vi "6. Module Attributes.vi"() -> ()   [LabVIEW 2017]
doc: "### 6. Module Attributes.vi\n\n#### Overview\n\nDemonstrates how to dynamically interact with CSM module attributes using VIs from outside the CSM framework.\n\n#### Introduction\n\nThis example demonstrates how to dynamically interact with CSM module attributes using VIs from outside the CSM framework.\n\nThe following are three ways of interaction within CSM framework:\n\n- Use string message queue to transfer message locally/outside of CSM framework, such as State >> Argument -@ DestModuleName.\n- Broadcast/Interrupt a status change event from a CSM module, register/unregister that event from another CSM/non-CSM module.\n- Use Module Attribute related VIs to get/set/remove/list CSM module attributes.\n\nThe core function of this example is from outside the CSM module to dynamically set another random number value to the CSM module, and then get the value from the CSM module and display the value on the UI.\n\n#### Steps\n\nStep 1: Drop the VI template from LabVIEW CSM palette.\n\nStep 2: Add one new line of state string after Macro:Initialize, namely API: Define ABC Attribute.\n\nStep 3: Set Module Attribute inside the CSM module: abc as attribute, a random number as value.\n\nStep 4: Set Module Attribute from outside the CSM module: abc as attribute, a random number as value.\n\nStep 5: Set Module Attribute from outside the CSM module: abc as attribute, retrieve the set random number as value.\n\nStep 6: Send a synchronous message to stop the CSM module from outside the CSM module."
uses:
  user.lib/_NEVSTOP/Communicable State Machine(CSM)/AdvanceAPI/CSM - Revert Arguments-Safe String.vi
  user.lib/_NEVSTOP/Communicable State Machine(CSM)/AdvanceAPI/CSM - Make String Arguments Safe.vi
  user.lib/_NEVSTOP/Communicable State Machine(CSM)/AdvanceAPI/CSM - Break Down Multiple States String.vi
  user.lib/_NEVSTOP/Communicable State Machine(CSM)/AdvanceAPI/CSM - Compact Multiple States.vi
  user.lib/_NEVSTOP/Communicable State Machine(CSM)/AdvanceAPI/CSM - Keywords.vi
  user.lib/_NEVSTOP/Communicable State Machine(CSM)/_Shared/Trim Single-line Text.vi
  user.lib/_NEVSTOP/Communicable State Machine(CSM)/Communicable State Machine.lvlib
panel:
  out "Waited(ms) 2":u32
  out "Waited(ms)":u32
  out "error out":errorcluster
  out "abc":dbl
  out "State History":string
  # "#CSM-Example Overview\n\nDemonstrates how to dynamically interact with CSM module attributes using VIs from outside the CSM framework."
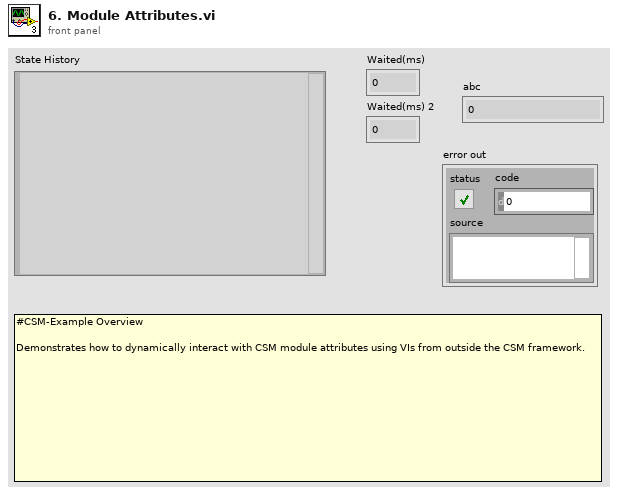
[diagram p1: front panel]
types:
  T1 = enum32{"Invalid", "Standard", "Closed", "Hidden", "Minimized", "Maximized"}
  T2 = enum32{"invalid app kind", "Development System", "Run Time System", "Student Edition", "Embedded LabVIEW", "Evaluation", "Custom"}
  T3 = typedef "Communicable State Machine.lvlib/_CSM_Response Source Message.ctl" = cluster{"‘State":string, "’Arguments":string, "’Error":errorcluster}
  T4 = cluster{"Current VI Reference":refnum<vi>, "Close Panel on Exit?":bool}
  T5 = cluster{"Core":cluster{"Current VI Reference":refnum<vi>, "Close Panel on Exit?":bool}, "Your Boolean data":bool, "Your string data":string}
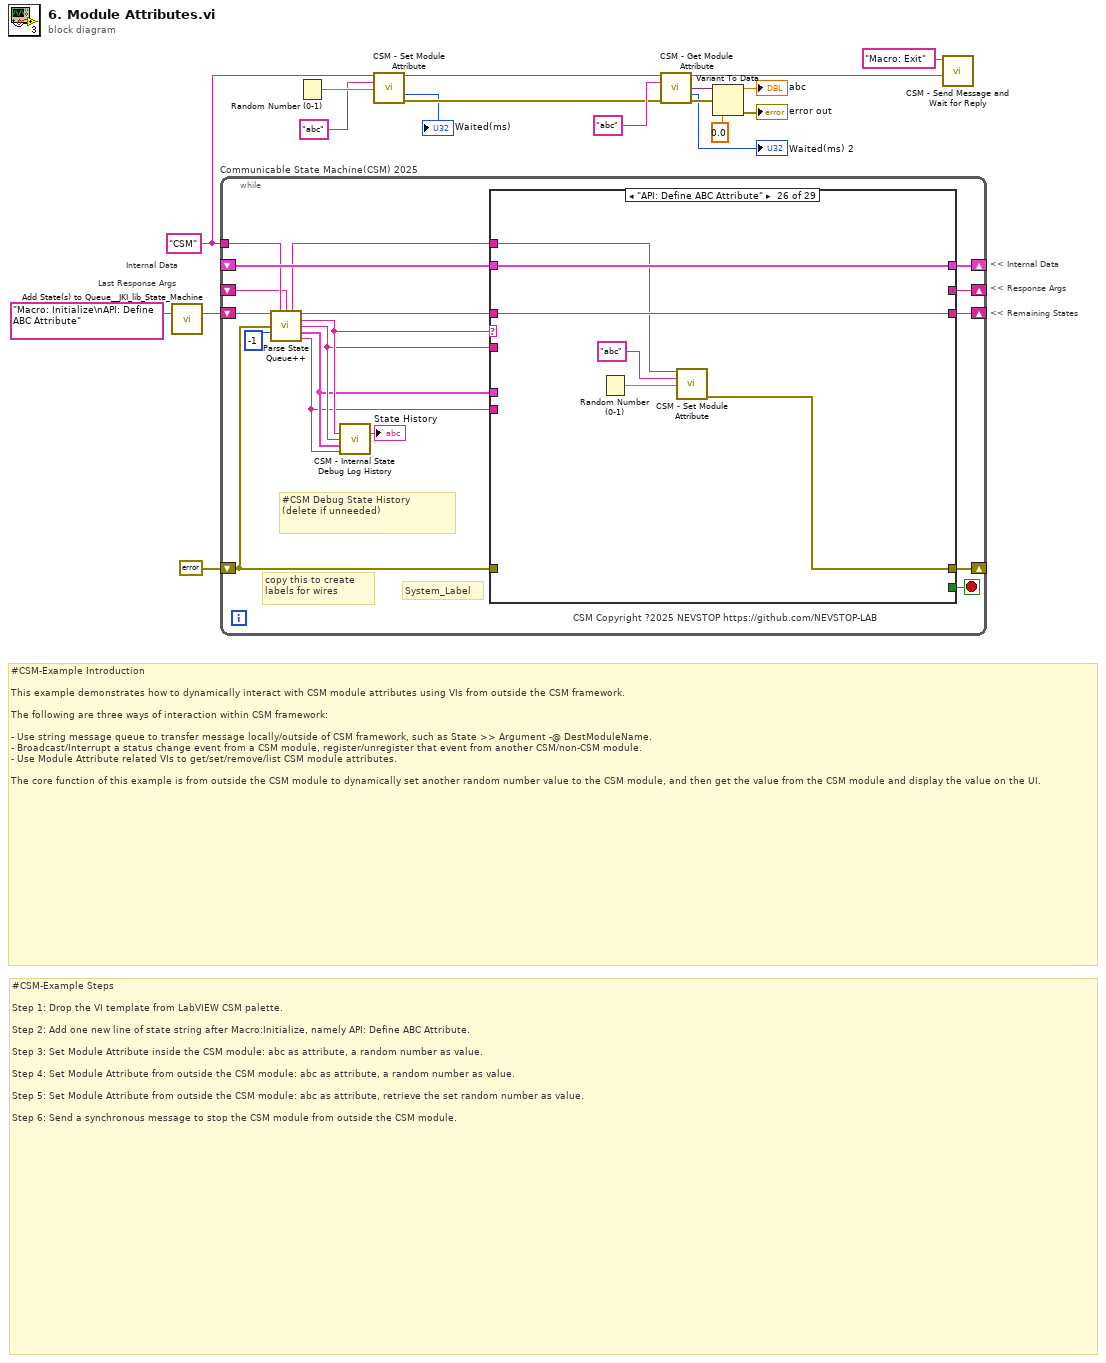
[diagram p0: block diagram]
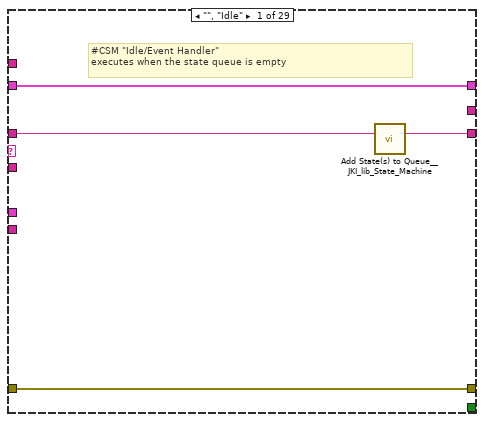
[diagram p2: hidden frame]
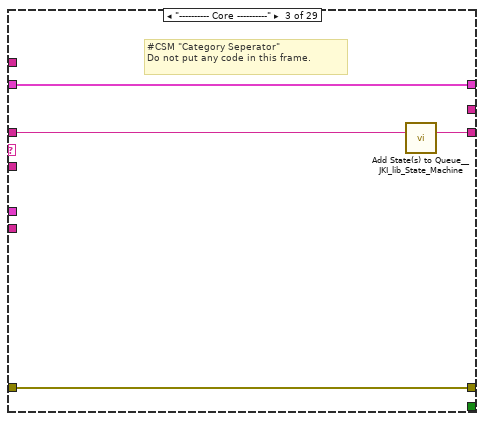
[diagram p4: hidden frame]
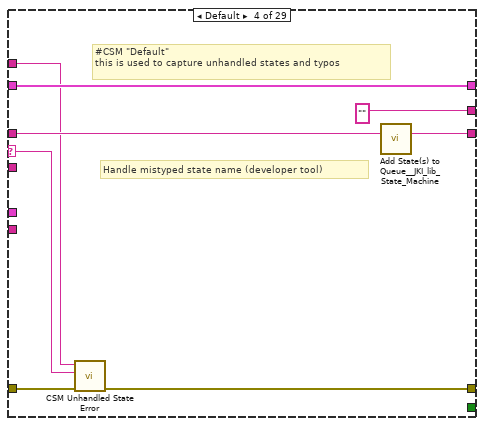
[diagram p5: hidden frame]
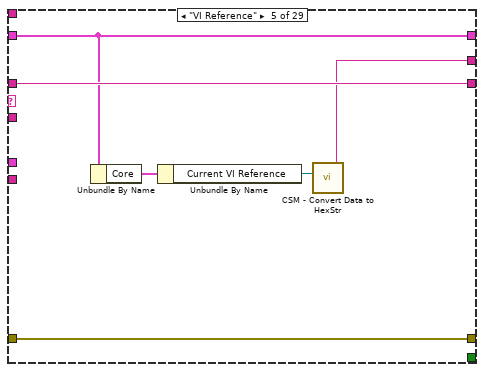
[diagram p6: hidden frame]
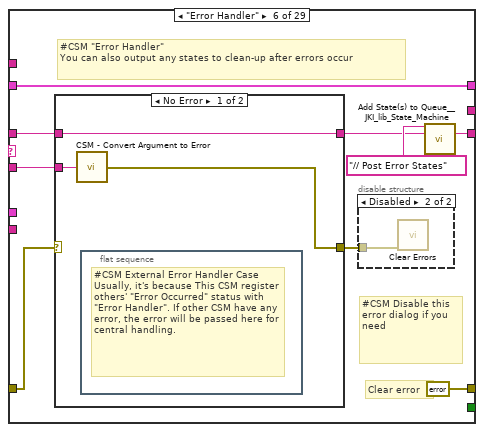
[diagram p7: hidden frame]
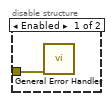
[diagram p8: hidden frame]
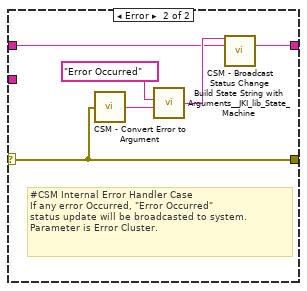
[diagram p9: hidden frame]
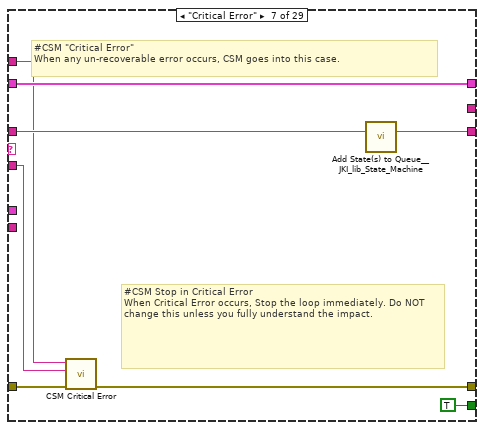
[diagram p10: hidden frame]
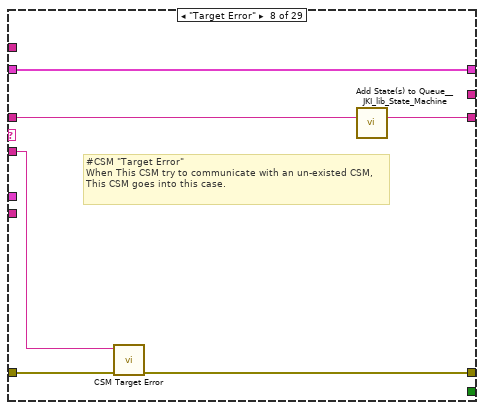
[diagram p11: hidden frame]
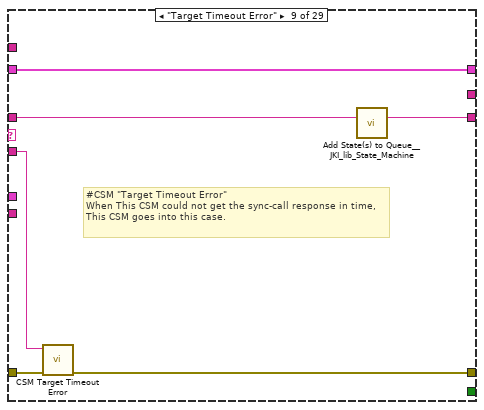
[diagram p12: hidden frame]
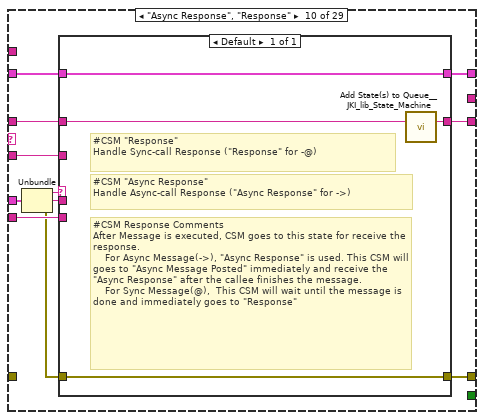
[diagram p13: hidden frame]
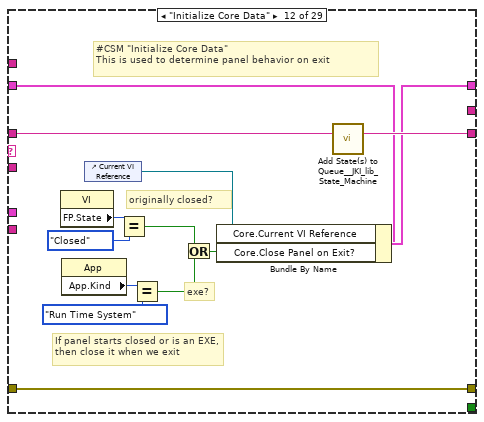
[diagram p15: hidden frame]
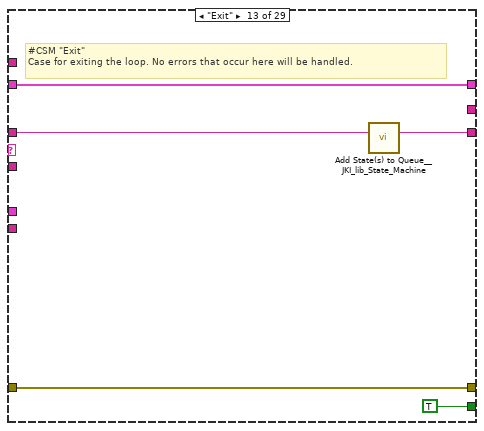
[diagram p16: hidden frame]
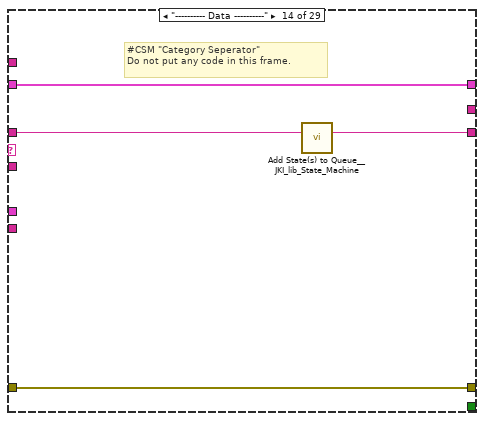
[diagram p17: hidden frame]
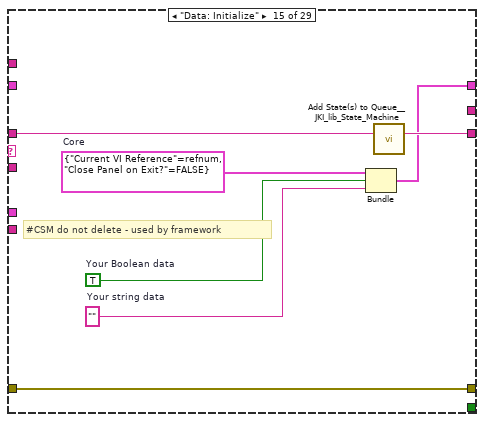
[diagram p18: hidden frame]
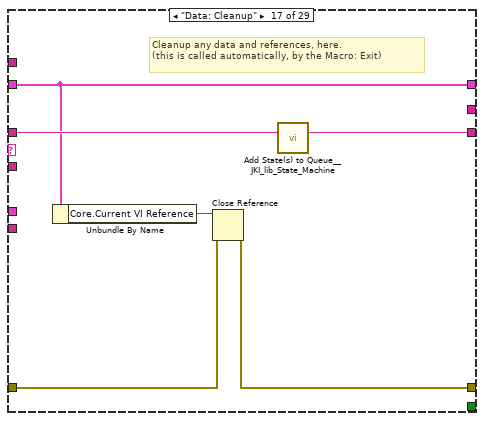
[diagram p20: hidden frame]
diagram:
  w3 = "CSM" ("Name(\"\" to use uuid)")
  # "#CSM-Example Steps\n\nStep 1: Drop the VI template from LabVIEW CSM palette.\n\nStep 2: Add one new line of state string after Macro:Initialize, namely API: Define ABC Attribute.\n\nStep 3: Set Module Attribute inside the CSM module: abc as attribute, a random number as value.\n\nStep 4: Set Module Attribute from outside the CSM module: abc as attribute, a random number as value.\n\nStep 5: Set Module Attribute from outside the CSM module: abc as attribute, retrieve the set random number as value.\n\nStep 6: Send a synchronous message to stop the CSM module from outside the CSM module."
  # "#CSM-Example Introduction\n\nThis example demonstrates how to dynamically interact with CSM module attributes using VIs from outside the CSM framework.\n\nThe following are three ways of interaction within CSM framework:\n\n- Use string message queue to transfer message locally/outside of CSM framework, such as State >> Argument -@ DestModuleName.\n- Broadcast/Interrupt a status change event from a CSM module, register/unregister that event from another CSM/non-CSM module.\n- Use Module Attribute related VIs to get/set/remove/list CSM module attributes.\n\nThe core function of this example is from outside the CSM module to dynamically set another random number value to the CSM module, and then get the value from the CSM module and display the value on the UI."
  # "Last Response Args"
  # "Internal Data"
  # "<< Internal Data"
  # "<< Response Args"
  # "<< Remaining States"
  n1 = call <vilib>:"Add State(s) to Queue__JKI_lib_State_Machine.vi"("State(s) in (\"\")"="Macro: Initialize\nAPI: Define ABC Attribute" ("Init State(\"Macro: Initialize\")")) -> ("States Out"=w16:string)  [unwired: 14 in]
  n2 = while "Communicable State Machine(CSM) 2025" {
    shift-right: [w31] -> _
    shift-left: _ -> [w30]
    shift-right: [w34] -> _
    shift-left: errorcluster {"status"=FALSE, "code"=0, "source"=""} ("error out") -> [w29]
    shift-right: [w33] -> _
    shift-left: w16 -> [w35]
    tunnel: w3 -> [w27]
    shift-right: [w28] -> _
    shift-left: _ -> [w21]
    stop <- w32 stop-if-true
    # "#CSM Debug State History\n(delete if unneeded)"
    # "copy this to create labels for wires"
    # "System_Label"
    # "CSM Copyright ?2025 NEVSTOP https://github.com/NEVSTOP-LAB"
    n3 = call "Parse State Queue++.vi"("State Queue"=w35, "Name (\"\" to Use UUID)"=w27, "Response Arguments"=w21, "Previous Error"=w29, "Dequeue (1 ms)"=-1 ("Timeout")) -> ("Name Used"=w22:string, "Remaining States"=w36:string, "Current State"=w26:string, "Arguments"=w25:string, ">> Response Source Message >>"=w24:T3, ">> Source CSM >>"=w23:string)  [unwired: 5 in]
    n4 = call "CSM - Internal State Debug Log History.vi"("State"=w26, "Arguments (\"\")"=w25, ">> Response Source Message >>"=w24, "Source (\"\")"=w23) -> ("Debug Log"=→"State History":string)  [unwired: 11 in]
    n5 = case shown="\"API: Define ABC Attribute\"" w26 {
      selector: w26 -> [_ _ _ w50 _ _ _ _ _ _ _ _ _ _ _ _ _ _ _ _ _ _ _ _ _ _ _ _ _]
      tunnel: w36 -> [w37 w42 w47 w54 w60 w66 w87 w93 w99 w107 w118 w132 w137 w141 w148 w150 w157 w161 w165 w171 w186 w255 w260 w267 w269 w276 w280 w284 w288]
      tunnel: w25 -> [_ _ _ _ _ w65 w83 w92 w97 w106 _ _ _ _ _ _ _ _ _ w166 w180 _ _ _ _ _ _ _ _]
      tunnel: w30 -> [w38 w41 w44 w52 w59 w69 w88 w94 w100 w109 w117 w125 w135 w138 _ w149 w152 w158 w163 w169 w182 w252 w257 w264 w268 w275 w277 w281 w285]
      tunnel: [w39 w43 w45 w48 w61 errorcluster {"status"=FALSE, "code"=0, "source"=""} ("error out") w84 w90 w96 w112 w119 w129 w134 w139 w145 w151 w153 w159 w162 w167 w183 w253 w258 w265 w270 w271 w278 w282 w286] -> w34
      tunnel: w29 -> [w39 w43 w45 w55 w61 w67 w89 w91 w98 _ w119 w129 w134 w139 w145 w151 w154 w159 w162 w168 w184 w253 w258 w265 w270 _ w278 w282 w286]
      tunnel: [w40 w42 w46 w53 w60 w62 w86 w95 w101 w108 w118 w131 w136 w140 w147 w150 w156 w160 w164 w170 w185 w254 w259 w266 w269 w276 w279 w283 w287] -> w33
      tunnel: [_ _ _ _ _ _ TRUE _ _ _ _ _ TRUE _ _ _ _ _ _ _ _ _ _ _ _ _ _ _ _] -> w32
      tunnel: [w38 w41 w44 w52 w59 w69 w88 w94 w100 w110 w117 w130 w135 w138 w146 w149 w152 w158 w163 w169 w182 w252 w257 w264 w268 w275 w277 w281 w285] -> w31
      tunnel: w23 -> [_ _ _ _ _ _ _ _ _ w104 _ _ _ _ _ _ _ _ _ _ _ _ _ _ _ _ _ _ _]
      tunnel: w24 -> [_ _ _ _ _ _ _ _ _ w111 _ _ _ _ _ _ _ _ _ _ _ _ _ _ _ _ _ _ _]
      tunnel: [_ _ _ "" w56 _ _ _ _ _ _ _ _ _ _ _ _ _ _ _ _ _ _ _ _ _ _ _ _] -> w28
      tunnel: w22 -> [_ _ _ w49 _ _ w82 _ _ _ _ _ _ _ _ _ _ _ _ _ _ _ _ _ _ w272 _ _ _]
      frame "", "Idle" {
        # "#CSM \"Idle/Event Handler\"\nexecutes when the state queue is empty"
        n6 = call <vilib>:"Add State(s) to Queue__JKI_lib_State_Machine.vi"("State(s) in (\"\")"=w37) -> ("States Out"=w40:string)  [unwired: 14 in]
      }
      frame "CSM Documentation" {
        # "#CSM README FIRST\n\nCommunicable State Machine(CSM) is a LabVIEW application framework that builds upon JKI State Machine(JKISM). It follows the pattern of JKISM and extends the keywords to describe message communication between modules, including concepts such as Sync-Message, Async-Message, Subscription/Unsubscription of status - essential elements for creating reusable code modules. For more information, please visit the CSM wiki: https://nevstop-lab.github.io/CSM-Wiki/\n\nFor instructions on JKI State Machine, visit: http://jki.net/state-machine/\nFor information about CSM, visit: https://github.com/NEVSTOP-LAB"
        # "#CSM \"Documentation\"\nCase for holding CSM Documenation"
      }
      frame "---------- Core ----------" {
        # "#CSM \"Category Seperator\"\nDo not put any code in this frame."
        n7 = call <vilib>:"Add State(s) to Queue__JKI_lib_State_Machine.vi"("State(s) in (\"\")"=w47) -> ("States Out"=w46:string)  [unwired: 14 in]
      }
      frame Default {
        # "#CSM \"Default\"\nthis is used to capture unhandled states and typos"
        # "Handle mistyped state name (developer tool)"
        n8 = call "CSM Unhandled State Error.vi"("error in (no error)"=w55, "Current State"=w50, "CSM Name"=w49) -> ("error out"=w48:errorcluster)  [unwired: 8 in]
        n9 = call <vilib>:"Add State(s) to Queue__JKI_lib_State_Machine.vi"("State(s) in (\"\")"=w54) -> ("States Out"=w53:string)  [unwired: 14 in]
      }
      frame "VI Reference" {
        n10 = Unbundle By Name(w59) -> ("Core"=w58:T4)
        n11 = Unbundle By Name(w58) -> ("Current VI Reference"=w57:refnum<vi>)
        n12 = call "CSM - Convert Data to HexStr.vi"("Variant"=w57) -> ("HEX String (0-9,A-F)"=w56:string)  [unwired: 8 in]
      }
      frame "Error Handler" {
        # "#CSM Disable this error dialog if you need"
        # "#CSM \"Error Handler\"\nYou can also output any states to clean-up after errors occur"
        # "Clear error"
        n13 = case shown="No Error" w67 {
          selector: w67 -> [_ w76]
          tunnel: [w75 w78] -> w63
          tunnel: w66 -> [w75 w77]
          tunnel: w65 -> [w74 _]
          tunnel: [w73 w76] -> w68
          frame No Error {
            n14 = call "CSM - Convert Argument to Error.vi"("Argument"=w74) -> ("Error"=w73:errorcluster)  [unwired: 4 in]
            n15 = flat-sequence {
              frame #0 {
                # "#CSM External Error Handler Case\nUsually, it's because This CSM register others' \"Error Occurred\" status with \"Error Handler\". If other CSM have any error, the error will be passed here for central handling."
              }
            }
          }
          frame Error {
            # "#CSM Internal Error Handler Case \nIf any error Occurred, \"Error Occurred\" \nstatus update will be broadcasted to system.\nParameter is Error Cluster."
            n16 = call "CSM - Convert Error to Argument.vi"("Error"=w76) -> ("Argument"=w80:string)  [unwired: 4 in]
            n17 = call <vilib>:"Build State String with Arguments__JKI_lib_State_Machine.vi"("Arguments (\"\")"=w80, "State"="Error Occurred" ("Status with Arguments")) -> ("State with Arguments"=w79:string)  [unwired: 4 in]
            n18 = call "CSM - Broadcast Status Change.vi"("Status With Arguments"=w79, "State Queue"=w77) -> ("Remaining States"=w78:string)  [unwired: 13 in]
          }
        }
        n19 = disable-structure shown="Disabled" {
          disable-tunnel: w68 -> [w71 w72]
          frame Enabled {
            n20 = call <vilib>:"General Error Handler.vi"("error in (no error)"=w71) -> ()  [unwired: 10 in, 5 out]
          }
          frame Disabled {
            n21 = call <vilib>:"Clear Errors.vi"("error in (no error)"=w72) -> ()  [unwired: 5 in, 2 out]
          }
        }
        n22 = call <vilib>:"Add State(s) to Queue__JKI_lib_State_Machine.vi"("State(s) in Front (\"\")"="// Post Error States", "State(s) in (\"\")"=w63) -> ("States Out"=w62:string)  [unwired: 13 in]
      }
      frame "Critical Error" {
        # "#CSM Stop in Critical Error\nWhen Critical Error occurs, Stop the loop immediately. Do NOT change this unless you fully understand the impact."
        # "#CSM \"Critical Error\"\nWhen any un-recoverable error occurs, CSM goes into this case."
        n23 = call "CSM Critical Error.vi"("error in (no error)"=w89, "Arugments (As Reason)"=w83, "CSM Name"=w82) -> ("error out"=w84:errorcluster)  [unwired: 8 in]
        n24 = call <vilib>:"Add State(s) to Queue__JKI_lib_State_Machine.vi"("State(s) in (\"\")"=w87) -> ("States Out"=w86:string)  [unwired: 14 in]
      }
      frame "Target Error" {
        # "#CSM \"Target Error\"\nWhen This CSM try to communicate with an un-existed CSM, This CSM goes into this case."
        n25 = call "CSM Target Error.vi"("error in (no error)"=w91, "Arguments (As CSM Name)"=w92) -> ("error out"=w90:errorcluster)  [unwired: 9 in]
        n26 = call <vilib>:"Add State(s) to Queue__JKI_lib_State_Machine.vi"("State(s) in (\"\")"=w93) -> ("States Out"=w95:string)  [unwired: 14 in]
      }
      frame "Target Timeout Error" {
        # "#CSM \"Target Timeout Error\"\nWhen This CSM could not get the sync-call response in time, This CSM goes into this case."
        n27 = call "CSM Target Timeout Error.vi"("error in (no error)"=w98, "Arguments (As CSM Name)"=w97) -> ("error out"=w96:errorcluster)  [unwired: 9 in]
        n28 = call <vilib>:"Add State(s) to Queue__JKI_lib_State_Machine.vi"("State(s) in (\"\")"=w99) -> ("States Out"=w101:string)  [unwired: 14 in]
      }
      frame "Async Response", "Response" {
        n29 = Unbundle(w111) -> ("‘State"=w105:string, "’Arguments"=w103:string, "’Error"=w102:errorcluster)
        n30 = case shown="Default" w105 {
          tunnel: [w116] -> w112
          tunnel: w102 -> [w116]
          tunnel: [w115] -> w110
          tunnel: w109 -> [w115]
          tunnel: [w113] -> w108
          tunnel: w107 -> [w114]
          tunnel: w106 -> [_]
          tunnel: w104 -> [_]
          tunnel: w103 -> [_]
          frame Default {
            # "#CSM Response Comments\nAfter Message is executed, CSM goes to this state for receive the response.\n    For Async Message(->), \"Async Response\" is used. This CSM will goes to \"Async Message Posted\" immediately and receive the \"Async Response\" after the callee finishes the message.\n    For Sync Message(@),  This CSM will wait until the message is done and immediately goes to \"Response\""
            # "#CSM \"Async Response\"\nHandle Async-call Response (\"Async Response\" for ->)"
            # "#CSM \"Response\"\nHandle Sync-call Response (\"Response\" for -@)"
            n31 = call <vilib>:"Add State(s) to Queue__JKI_lib_State_Machine.vi"("State(s) in (\"\")"=w114) -> ("States Out"=w113:string)  [unwired: 14 in]
          }
        }
      }
      frame "Async Message Posted" {
        # "#CSM \"Async Message Posted\"\nAfter Async Message is posted (-> or ->| ), CSM goes to this state for post-action.\nYou can use Argument - State to tell which Async Message is called."
      }
      frame "Initialize Core Data" {
        # "#CSM \"Initialize Core Data\"\nThis is used to determine panel behavior on exit"
        # "originally closed?"
        # "exe?"
        # "If panel starts closed or is an EXE, then close it when we exit"
        n32 = property class="VI"() -> ("FP.State"=w122:T1)  [unwired: 2 in, 2 out]
        n33 = property class="App"() -> ("App.Kind"=w128:T2)  [unwired: 2 in, 2 out]
        n34 = control-ref of="Current VI Reference"() -> (w123:refnum<vi>)
        n35 = Equal?(x=w122, y=T1."Closed" ("Front Panel Window:State")) -> (x = y?=w120:bool)
        n36 = Equal?(x=w128, y=T2."Run Time System" ("Application:Kind")) -> (x = y?=w126:bool)
        n37 = Or(x=w120, y=w126) -> (x .or. y?=w124:bool)
        n38 = Bundle By Name(cluster=w125, "Core.Current VI Reference"=w123, "Core.Close Panel on Exit?"=w124) -> (w130:T5)
        n39 = call <vilib>:"Add State(s) to Queue__JKI_lib_State_Machine.vi"("State(s) in (\"\")"=w132) -> ("States Out"=w131:string)  [unwired: 14 in]
      }
      frame "Exit" {
        # "#CSM \"Exit\"\nCase for exiting the loop. No errors that occur here will be handled."
        n40 = call <vilib>:"Add State(s) to Queue__JKI_lib_State_Machine.vi"("State(s) in (\"\")"=w137) -> ("States Out"=w136:string)  [unwired: 14 in]
      }
      frame "---------- Data ----------" {
        # "#CSM \"Category Seperator\"\nDo not put any code in this frame."
        n41 = call <vilib>:"Add State(s) to Queue__JKI_lib_State_Machine.vi"("State(s) in (\"\")"=w141) -> ("States Out"=w140:string)  [unwired: 14 in]
      }
      frame "Data: Initialize" {
        w142 = T4 {"Current VI Reference"=refnum, "Close Panel on Exit?"=FALSE}  # Core
        w144 = TRUE  # Your Boolean data
        w143 = ""  # Your string data
        # "#CSM do not delete - used by framework"
        n42 = Bundle("Core"=w142, "Your Boolean data"=w144, "Your string data"=w143) -> (w146:T5)  [unwired: 1 in]
        n43 = call <vilib>:"Add State(s) to Queue__JKI_lib_State_Machine.vi"("State(s) in (\"\")"=w148) -> ("States Out"=w147:string)  [unwired: 14 in]
      }
      frame "Data: Update Indicators" {
      }
      frame "Data: Cleanup" {
        # "Cleanup any data and references, here.\n(this is called automatically, by the Macro: Exit)"
        n44 = Unbundle By Name(w152) -> ("Core.Current VI Reference"=w155:refnum<vi>)
        n45 = Close Reference(reference=w155, error in (no error)=w154) -> (error out=w153:errorcluster)
        n46 = call <vilib>:"Add State(s) to Queue__JKI_lib_State_Machine.vi"("State(s) in (\"\")"=w157) -> ("States Out"=w156:string)  [unwired: 14 in]
      }
      frame "---------- UI ----------" {
        # "#CSM \"Category Seperator\"\nDo not put any code in this frame."
        n47 = call <vilib>:"Add State(s) to Queue__JKI_lib_State_Machine.vi"("State(s) in (\"\")"=w161) -> ("States Out"=w160:string)  [unwired: 14 in]
      }
      frame "UI: Initialize" {
        # "#CSM \"UI: Initialize\"\nInitialize the User Interface, here.\n(this is called automatically, by the Macro: Init)"
        n48 = call <vilib>:"Add State(s) to Queue__JKI_lib_State_Machine.vi"("State(s) in (\"\")"=w165) -> ("States Out"=w164:string)  [unwired: 14 in]
      }
      frame "UI: Cursor Set" {
        # "#CSM \"UI: Cursor Set\"\nSet and Unset Cursor Busy.\n(Usage: \"UI: Cursor Set >> Busy|Idle\")"
        # "Argument"
        n49 = disable-structure shown="TARGET_TYPE!=Windows" {
          disable-tunnel: w168 -> [w174 w179]
          disable-tunnel: [w173 w179] -> w167
          disable-tunnel: w166 -> [w172 _]
          frame condition #0 (active) {
            n50 = case shown="\"Idle\", Default" w172 {
              tunnel: w174 -> [w176 w178]
              tunnel: [w175 w177] -> w173
              frame "Idle", Default {
                n51 = call <vilib>:"Unset Busy.vi"("error in (no error)"=w176) -> ("error out"=w175:errorcluster)  [unwired: 10 in]
              }
              frame "Busy" {
                n52 = call <vilib>:"Set Busy.vi"("error in (no error)"=w178) -> ("error out"=w177:errorcluster)  [unwired: 9 in, 1 out]
              }
            }
          }
          frame condition #1 {
          }
        }
        n53 = call <vilib>:"Add State(s) to Queue__JKI_lib_State_Machine.vi"("State(s) in (\"\")"=w171) -> ("States Out"=w170:string)  [unwired: 14 in]
      }
      frame "UI: Front Panel State" {
        # "#CSM \"UI: Front Panel State\"\nSet Front Panel Open or Closed\n(Usage: \"UI: Front Panel State >> Open|Close\")"
        # "Argument"
        n54 = Unbundle By Name(w182) -> ("Core.Current VI Reference"=w181:refnum<vi>)
        n55 = call <vilib>:"Add State(s) to Queue__JKI_lib_State_Machine.vi"("State(s) in (\"\")"=w186) -> ("States Out"=w185:string)  [unwired: 14 in]
        n56 = case shown="\"Close\", \"Closed\"" w180 {
          tunnel: w184 -> [w192 w207 w218 w231 w244]
          tunnel: [w194 w208 w220 w233 w246] -> w183
          tunnel: w181 -> [w193 w205 w219 w232 w245]
          frame "Open", "Standard", Default {
            w187 = T1."Standard" ("State")
            n57 = property class="VI"(reference=w193, error in=w192) -> (reference out=w190:refnum<vi>, error out=w191:errorcluster, "FP.State"=w189:T1)
            n58 = Not Equal?(x=w189, y=w187) -> (x != y?=w188:bool)
            n59 = case shown="True" w188 {
              tunnel: [w198 w200] -> w194
              tunnel: w191 -> [w197 w200]
              tunnel: w190 -> [w196 _]
              tunnel: w187 -> [w195 _]
              frame True {
                n60 = invoke class="VI" method="FP.Open"(reference=w196, error in=w197, "Activate"=TRUE, "State"=w195) -> (error out=w198:errorcluster)  [unwired: 1 in, 4 out]
              }
              frame False {
              }
            }
          }
          frame "Close", "Closed" {
            n61 = property class="VI"(reference=w205, error in=w207) -> (reference out=w204:refnum<vi>, error out=w206:errorcluster, "FP.State"=w202:T1)
            n62 = Not Equal?(x=w202, y=T1."Closed" ("Front Panel Window:State")) -> (x != y?=w201:bool)
            n63 = case shown="False" w201 {
              tunnel: [w209 w212] -> w208
              tunnel: w206 -> [w209 w211]
              tunnel: w204 -> [_ w210]
              frame False {
              }
              frame True {
                n64 = invoke class="VI" method="FP.Close"(reference=w210, error in=w211) -> (error out=w212:errorcluster)  [unwired: 1 in, 2 out]
              }
            }
          }
          frame "Hidden", "Hide" {
            w213 = T1."Hidden" ("State")
            n65 = property class="VI"(reference=w219, error in=w218) -> (reference out=w216:refnum<vi>, error out=w217:errorcluster, "FP.State"=w215:T1)
            n66 = Not Equal?(x=w215, y=w213) -> (x != y?=w214:bool)
            n67 = case shown="True" w214 {
              tunnel: [w224 w225] -> w220
              tunnel: w217 -> [w223 w225]
              tunnel: w216 -> [w222 _]
              tunnel: w213 -> [w221 _]
              frame True {
                n68 = invoke class="VI" method="FP.Open"(reference=w222, error in=w223, "State"=w221) -> (error out=w224:errorcluster)  [unwired: 2 in, 4 out]
              }
              frame False {
              }
            }
          }
          frame "Minimize", "Minimized" {
            w226 = T1."Minimized" ("State")
            n69 = property class="VI"(reference=w232, error in=w231) -> (reference out=w229:refnum<vi>, error out=w230:errorcluster, "FP.State"=w228:T1)
            n70 = Not Equal?(x=w228, y=w226) -> (x != y?=w227:bool)
            n71 = case shown="True" w227 {
              tunnel: [w237 w238] -> w233
              tunnel: w230 -> [w236 w238]
              tunnel: w229 -> [w235 _]
              tunnel: w226 -> [w234 _]
              frame True {
                n72 = invoke class="VI" method="FP.Open"(reference=w235, error in=w236, "State"=w234) -> (error out=w237:errorcluster)  [unwired: 2 in, 4 out]
              }
              frame False {
              }
            }
          }
          frame "Maximize", "Maximized" {
            w239 = T1."Maximized" ("State")
            n73 = property class="VI"(reference=w245, error in=w244) -> (reference out=w242:refnum<vi>, error out=w243:errorcluster, "FP.State"=w241:T1)
            n74 = Not Equal?(x=w241, y=w239) -> (x != y?=w240:bool)
            n75 = case shown="True" w240 {
              tunnel: [w250 w251] -> w246
              tunnel: w243 -> [w249 w251]
              tunnel: w242 -> [w248 _]
              tunnel: w239 -> [w247 _]
              frame True {
                n76 = invoke class="VI" method="FP.Open"(reference=w248, error in=w249, "State"=w247) -> (error out=w250:errorcluster)  [unwired: 2 in, 4 out]
              }
              frame False {
              }
            }
          }
        }
      }
      frame "---------- Macro ----------" {
        # "#CSM \"Category Seperator\"\nDo not put any code in this frame."
        n77 = call <vilib>:"Add State(s) to Queue__JKI_lib_State_Machine.vi"("State(s) in (\"\")"=w255) -> ("States Out"=w254:string)  [unwired: 14 in]
      }
      frame "Macro: Initialize" {
        # "#CSM \"Macro: Initialize\"\nInitialization Macro (This is called once, when the VI starts)"
        n78 = call <vilib>:"Add State(s) to Queue__JKI_lib_State_Machine.vi"("State(s) in Front (\"\")"="Data: Initialize\nInitialize Core Data\nData: Update Indicators", "State(s) in (\"\")"=w260) -> ("States Out"=w259:string)  [unwired: 13 in]
      }
      frame "Macro: Exit" {
        # "#CSM \"Macro: Exit\"\nExit Macro (This is called once, when the VI exits)"
        n79 = call <vilib>:"Add State(s) to Queue__JKI_lib_State_Machine.vi"("State(s) in Front (\"\")"="//Exit Sub-Modules ", "State(s) at Back (\"\")"="Data: Cleanup\nExit") -> ("States Out"=w262:string)  [unwired: 13 in]
        n80 = call <vilib>:"Add State(s) to Queue__JKI_lib_State_Machine.vi"("State(s) in Front (\"\")"=w262, "State(s) in (\"\")"=w267) -> ("States Out"=w266:string)  [unwired: 13 in]
      }
      frame "---------- API ----------" {
        # "#CSM \"Category Seperator\"\nDo not put any code in this frame."
      }
      frame "API: Define ABC Attribute" {
        n81 = Random Number (0-1)() -> (number: 0 to 1=w274:dbl)
        n82 = call "CSM - Set Module Attribute.vi"("CSM Name"=w272, "Attribute"="abc", "Value"=w274) -> ("error out"=w271:errorcluster)  [unwired: 9 in, 3 out]
      }
      frame "---------- Action ----------" {
        # "#CSM \"Category Seperator\"\nDo not put any code in this frame."
        n83 = call <vilib>:"Add State(s) to Queue__JKI_lib_State_Machine.vi"("State(s) in (\"\")"=w280) -> ("States Out"=w279:string)  [unwired: 14 in]
      }
      frame "Action: action1" {
        # "#CSM \"Internal State\"\nThis category is used for holding internal states"
        n84 = call <vilib>:"Add State(s) to Queue__JKI_lib_State_Machine.vi"("State(s) in (\"\")"=w284) -> ("States Out"=w283:string)  [unwired: 14 in]
      }
      frame "Action: action2" {
        # "#CSM \"Internal State\"\nThis category is used for holding internal states"
        n85 = call <vilib>:"Add State(s) to Queue__JKI_lib_State_Machine.vi"("State(s) in (\"\")"=w288) -> ("States Out"=w287:string)  [unwired: 14 in]
      }
    }
  }
  n86 = Random Number (0-1)() -> (number: 0 to 1=w7:dbl)
  n87 = call "CSM - Set Module Attribute.vi"("CSM Name"=w3, "Attribute"="abc", "Value"=w7) -> ("CSM Name (Dup)"=w4:string, "Waited (ms)"=→"Waited(ms)":u32, "error out"=w5:errorcluster)  [unwired: 9 in, 1 out]
  n88 = call "CSM - Get Module Attribute.vi"("CSM Name"=w4, "Attribute"="abc", "Error In"=w5) -> ("CSM Name (Dup)"=w10:string, "Value"=w13:variant, "Waited (ms)"=→"Waited(ms) 2":u32, "error out"=w14:errorcluster)  [unwired: 8 in, 1 out]
  n89 = Variant To Data(error in=w14, type=0.0, Variant=w13) -> (data=→"abc":dbl, error out=→"error out":errorcluster)
  n90 = call "CSM - Send Message and Wait for Reply.vi"("Target Module"=w10, "State"="Macro: Exit") -> ()  [unwired: 7 in, 3 out]
